vi "Write Ctl Refnum.vi"(8 "error in (no error)":errorcluster, 10 "Ctl Refnum":refnum<vi>, 11 "Field in":refnum<class "Field.lvclass">) -> (0 "error out":errorcluster, 3 "Field out":refnum<class "Field.lvclass">)   [LabVIEW 2020, in "Field.lvlib" / "Field.lvclass"]
uses:
  Field.lvclass
  Field.lvclass/Field.ctl
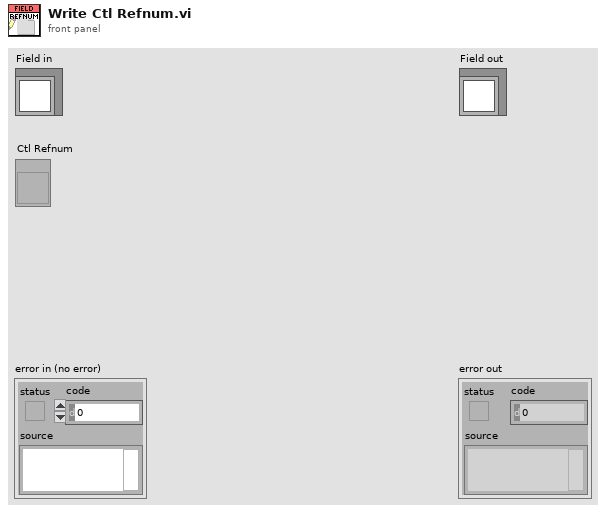
[diagram p1: front panel]
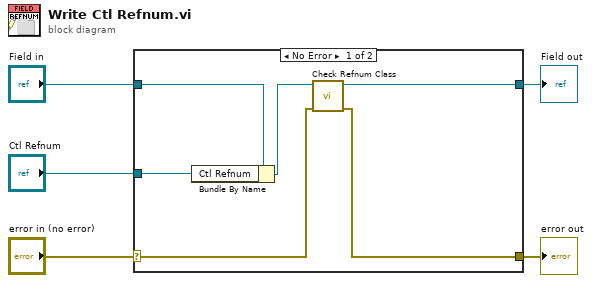
[diagram p0: block diagram]
diagram:
  n1 = case shown="No Error" "error in (no error)" {
    selector: "error in (no error)" -> [w7 w12]
    tunnel: [w6 w12] -> w4
    tunnel: [w8 w13] -> w2
    tunnel: "Field in" -> [w11 w13]
    tunnel: "Ctl Refnum" -> [w10 _]
    frame No Error {
      n2 = Bundle By Name(cluster=w11, "Ctl Refnum"=w10) -> (w9:refnum<class "Field.lvclass">)
      n3 = call-dynamic "Check Refnum Class.vi"("error in (no error)"=w7, "Field in"=w9) -> ("error out"=w6:errorcluster, "Field out"=w8:refnum<class "Field.lvclass">)  [unwired: 8 in]
    }
    frame Error {
    }
  }
  "error out" <- w4
  "Field out" <- w2
